vi "ConfigureDOforDcamHelper.vi"(0 "object in":refnum<class "AD2_SDK.lvclass">, 2 "Pulse Settings":T1, 5 "error in (no error)":errorcluster) -> (14 "object out":refnum<class "AD2_SDK.lvclass">, 19 "error out":errorcluster)   [LabVIEW 2021, in "AD2_SDK.lvclass"]
uses:
  AD2_SDK.lvclass
  AD2_SDK.lvclass/AD2_SDK.ctl
  AD2_DO_SDK_class/AD2_DO_SDK.lvclass
panel:
  # "DIO0 Pulses at the same time as DIO1,2 and 3 +-offset"
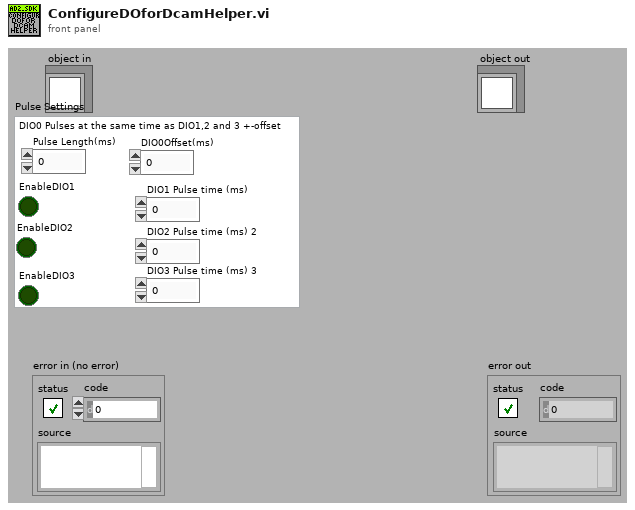
[diagram p1: front panel]
types:
  T1 = cluster{"Pulse Length(ms)":dbl, "DIO0Offset(ms)":dbl, "DIO1 Pulse time (ms)":dbl, "DIO2 Pulse time (ms) 2":dbl, "DIO3 Pulse time (ms) 3":dbl, "EnableDIO3":bool, "EnableDIO2":bool, "EnableDIO1":bool}
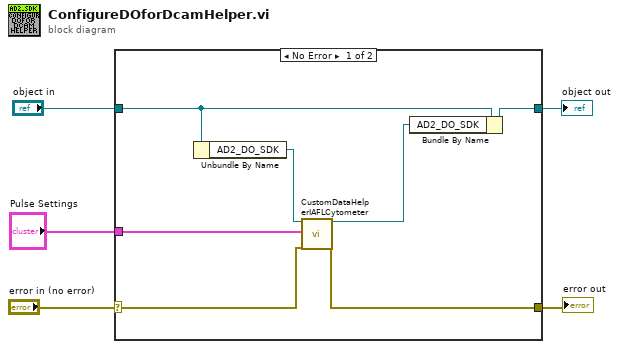
[diagram p0: block diagram]
diagram:
  n1 = case shown="No Error" "error in (no error)" {
    selector: "error in (no error)" -> [w8 w14]
    tunnel: [w7 w14] -> w4
    tunnel: [w10 w13] -> w2
    tunnel: "object in" -> [w12 w13]
    tunnel: "Pulse Settings" -> [w6 _]
    frame No Error {
      n2 = Unbundle By Name(w12) -> ("AD2_DO_SDK"=w11:refnum<class "AD2_DO_SDK.lvclass">)
      n3 = call-dynamic "CustomDataHelperIAFLCytometer.vi"("object in"=w11, "Pulse Settings"=w6, "error in (no error)"=w8) -> ("object out"=w9:refnum<class "AD2_DO_SDK.lvclass">, "error out"=w7:errorcluster)  [unwired: 15 in]
      n4 = Bundle By Name(cluster=w12, "AD2_DO_SDK"=w9) -> (w10:refnum<class "AD2_SDK.lvclass">)
    }
    frame Error {
    }
  }
  "error out" <- w4
  "object out" <- w2
